vi "CDO Configuration to Channel Settings.vi"(6 "CDO":T3, 8 "error in":errorcluster, 9 "default values":dbl[](array[numeric]), 10 "names":string[](array[string]), 11 "Counter Driven Output Mode in":refnum<class "Counter Driven Output Mode.lvclass">) -> (0 "error out":errorcluster, 1 "channel settings":T1[](array[typedef]), 2 "drive from slot":u32, 3 "Counter Driven Output Mode out":refnum<class "Counter Driven Output Mode.lvclass">)   [LabVIEW 2017, in "Scan Engine Scripting.lvlib" / "Counter Driven Output Mode.lvclass"]
uses:
  Counter Driven Output Mode.lvclass
  Controls/counter driven output channel settings.ctl
  Channel Classes/Counter Driven Output Channel/Counter Driven State.ctl
  Channel Classes/Counter Driven Output Channel/Counter Driven Output Channel.lvclass
  Scan Engine Scripting.lvlib
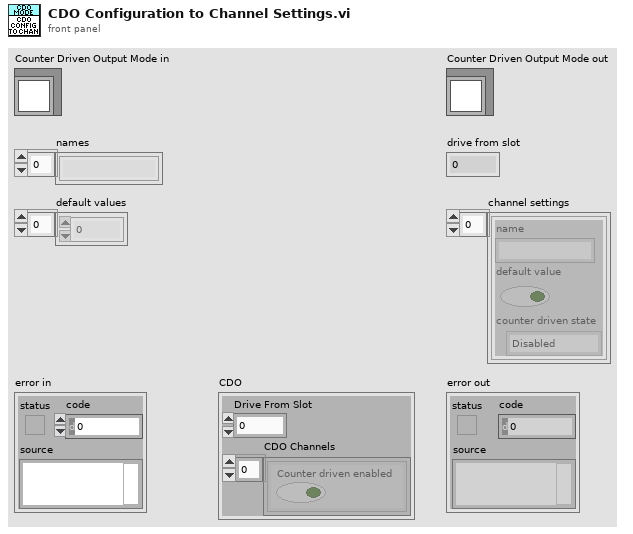
[diagram p1: front panel]
types:
  T1 = typedef "Scan Engine Scripting.lvlib/counter driven output channel settings.ctl" = cluster{"name":string, "default value":bool, "counter driven state":T2}
  T2 = typedef "Scan Engine Scripting.lvlib/Counter Driven Output Channel.lvclass/Counter Driven State.ctl" = enum16{"Disabled", "Enabled"}
  T3 = cluster{"Drive From Slot":u32, "CDO Channels":cluster{"Counter driven enabled":bool}[]}
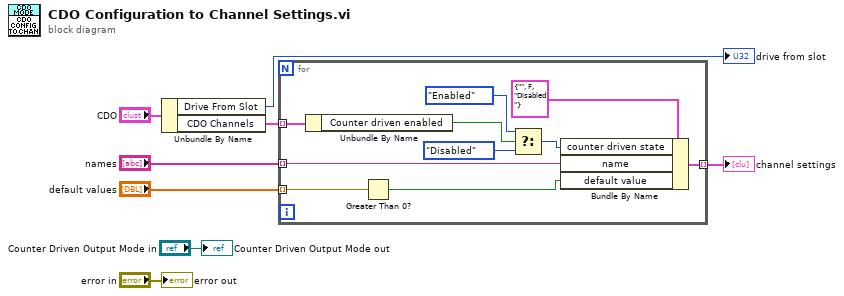
[diagram p0: block diagram]
diagram:
  n1 = Unbundle By Name("CDO") -> ("Drive From Slot"=→"drive from slot":u32, "CDO Channels"=w8:cluster{"Counter driven enabled":bool}[])
  n2 = for {
    tunnel: w8 -> [w18] mode=indexing
    tunnel: [w16] -> w5 mode=indexing
    tunnel: "names" -> [w11] mode=indexing
    tunnel: "default values" -> [w10] mode=indexing
    n3 = Unbundle By Name(w18) -> ("Counter driven enabled"=w13:bool)
    n4 = Greater Than 0?(x=w10) -> (x > 0?=w9:bool)
    n5 = Select(t=Counter_Driven_State."Enabled" ("counter driven state"), s=w13, f=Counter_Driven_State."Disabled" ("counter driven state")) -> (s? t:f=w12:T2)
    n6 = Bundle By Name(cluster=T1 {"name"="", "default value"=FALSE, "counter driven state"=enum."Disabled"} ("channel settings"), "counter driven state"=w12, "name"=w11, "default value"=w9) -> (w16:T1)
  }
  "channel settings" <- w5
  "error out" <- "error in"
  "Counter Driven Output Mode out" <- "Counter Driven Output Mode in"
